vi "Get Picture.vi"(8 "error in (no error)":errorcluster, 11 "Pulseblaster in":refnum<class "Slave_Pulseblaster.lvclass">) -> (0 "error out":errorcluster, 2 "Device Pic":T1, 3 "Pulseblaster out":refnum<class "Slave_Pulseblaster.lvclass">)   [LabVIEW 2013, in "Slave_Pulseblaster.lvclass"]
uses:
  Slave_Pulseblaster.lvclass
  <vilib>/picture/picture.llb/imagedata.ctl
panel:
  in  "Filename":string="slave_pulseblaster.png"
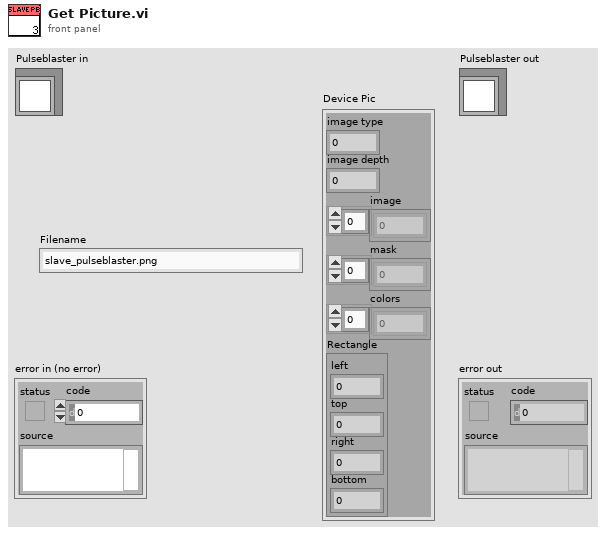
[diagram p1: front panel]
types:
  T1 = typedef "imagedata.ctl" = cluster{"image type":i32, "image depth":i32, "image":u8[], "mask":u8[], "colors":u32[], "Rectangle":cluster{"left":i16, "top":i16, "right":i16, "bottom":i16}}
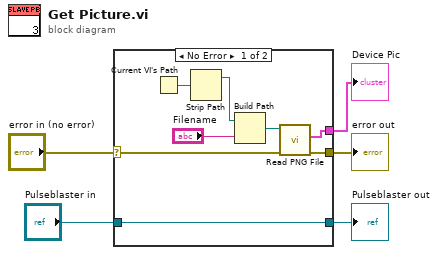
[diagram p0: block diagram]
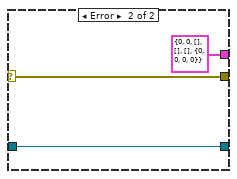
[diagram p2: hidden frame]
diagram:
  n1 = case shown="No Error" "error in (no error)" {
    selector: "error in (no error)" -> [w12 w16]
    tunnel: [w11 w16] -> w2
    tunnel: [w13 w15] -> w3
    tunnel: "Pulseblaster in" -> [w13 w15]
    tunnel: [w10 T1 {"image type"=0, "image depth"=0, "image"=[], "mask"=[], "colors"=[], "Rectangle"={"left"=0, "top"=0, "right"=0, "bottom"=0}} ("image data")] -> w1
    frame No Error {
      n2 = Current VI's Path() -> (path=w9:path)
      n3 = Strip Path(path=w9) -> (stripped path=w8:path)  [unwired: 1 out]
      n4 = Build Path(base path=w8, name or relative path="Filename") -> (appended path=w6:path)
      n5 = call <vilib>:"Read PNG File.vi"("error in (no error)"=w12, "path to PNG file"=w6) -> ("error out"=w11:errorcluster, "image data"=w10:T1)  [unwired: 7 in, 1 out]
    }
    frame Error {
    }
  }
  "error out" <- w2
  "Pulseblaster out" <- w3
  "Device Pic" <- w1
